vi "Copy_eID_Image.vi"(6 "eID_Details":T1, 11 "Image Location":path) -> ()   [LabVIEW 2020]
uses:
  Controls/user_log.ctl
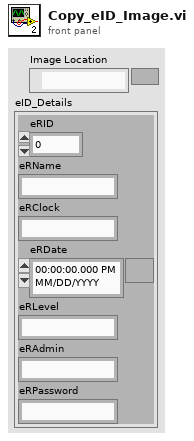
[diagram p1: front panel]
types:
  T1 = typedef "user_log.ctl" = cluster{"eRID":u16, "eRName":string, "eRClock":string, "eRDate":timestamp, "eRLevel":string, "eRAdmin":string, "eRPassword":string}
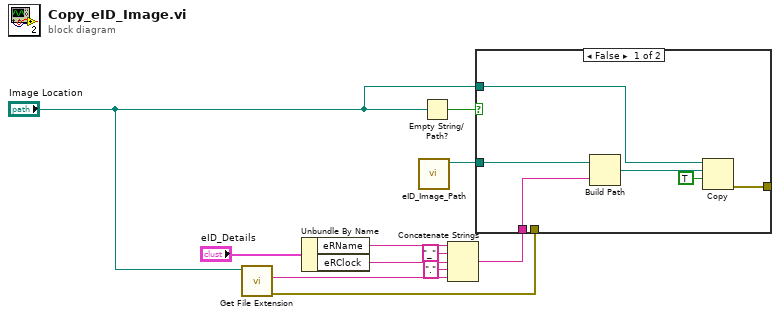
[diagram p0: block diagram]
diagram:
  n1 = call <vilib>:"Get File Extension.vi"("file"="Image Location") -> ("error out"=w1:errorcluster, "lowercase file extension"=w3:string)  [unwired: 6 in, 3 out]
  n2 = Unbundle By Name("eID_Details") -> ("eRName"=w8:string, "eRClock"=w7:string)
  n3 = call "eID_Image_Path.vi"() -> ("Path out"=w10:path)  [unwired: 11 in]
  n4 = Empty String/Path?(string/path="Image Location") -> (empty?=w11:bool)
  n5 = Concatenate Strings(w8, "_" ("string"), w7, "." ("string"), w3) -> (w5:string)
  n6 = case shown="False" w11 {
    tunnel: "Image Location" -> [w14 _]
    tunnel: w10 -> [w17 _]
    tunnel: w5 -> [w16 _]
    tunnel: w1 -> [_ _]
    tunnel: [w12 _] -> _
    frame False {
      n7 = Build Path(base path=w17, name or relative path=w16) -> (appended path=w15:path)
      n8 = Copy(9:TRUE ("overwrite (F)"), 10:w15, 11:w14) -> (0:w12:errorcluster)  [unwired: 2 in, 2 out]
    }
    frame True {
    }
  }
